vi "svx_Build Data from Magnitude and Phase (N Orders).vi"(5 "reset? (F)":bool, 6 "samples/revolution wanted":i32=4, 7 "samples/revolution":dbl=1.0 format="%.2f", 8 "error in (no error)":errorcluster, 9 "magnitudes info":T1[](array[typedef]) {"x-axis units" items=["Time (s)"=0, "Frequency-CB (Hz)"=1, "Frequency-CPB (Hz)"=1248, "Frequency-Arbitrary (Hz)"=2357, "Quefrency (s)"=2, "Revolutions (rev)"=3, "Order"=4, "Speed (RPM)"=11, "Speed (rad/s)"=21, "Index"=65535]; "weighting filter" items=["Linear", "A-weighting", "B-weighting", "C-weighting", "ITU-R 468-4", "Dolby", "CCITT", "C-message", "Wb", "Wc", "Wd", "We", "Wf", "Wh", "Wj", "Wk", "Wm", "AES17 20 kHz lowpass", "AES17 40 kHz lowpass", "AES17 20 kHz highpass", "AES17 40 kHz highpass"]; "dB reference [EU]" format="%.2f"; "engineering units" items=["custom..."=0, "V"=1, "A"=21, "C"=30, "pC"=31, "s"=32, "-"=29, "Pa"=2, "N"=20, "g"=3, "m/s^2"=4, "m/s"=5, "m"=6, "mm/s"=12, "mm"=13, "micron/s"=14, "micron"=15, "in/s^2"=7, "in/s"=8, "in"=9, "mil/s"=10, "mil"=11, "rad/s^2"=16, "rad/s"=17, "rad"=18, "deg/s^2"=26, "deg/s"=27, "deg"=28, "RPM"=22, "cycle/s^2"=23, "Hz"=24, "cycle"=25, "strain"=19]; "spectral info"."window" items=["None "=0, "Hanning"=1, "Hamming"=2, "Blackman-Harris"=3, "Exact Blackman"=4, "Blackman"=5, "Flat Top"=6, "4 Term B-Harris "=7, "7 Term B-Harris"=8, "Low Sidelobe"=9, "Force - Exponential"=10, "Gaussian"=62]}, 10 "phases [phase lag]":cluster{"time/rev/rpm":dbl[], "phase":dbl[]}[][](array[cluster]) {"phase" format="%.2f"; "time/rev/rpm" format="%.2f"}, 11 "magnitudes [RMS]":T7(array[cluster]) {"magnitude" format="%.2f"; "time/rev/rpm" format="%.2f"}) -> (0 "error out":errorcluster, 2 "actual samples/rev":dbl, 3 "order data":dbl[][][](array[numeric]), 4 "orders to compute":dbl[](array[numeric]))   [LabVIEW 2017]
uses:
  <vilib>/addons/_NISVFA/_Shared subVIs/Controls/svc_Spectrum Info.ctl
  <vilib>/addons/_NISVFA/_Shared subVIs/Controls/svc_X-Axis Units.ctl
  <vilib>/addons/_NISVFA/_Shared subVIs/Controls/svc_Spectrum Type.ctl
  <vilib>/addons/_NISVFA/_Shared subVIs/Controls/svc_Engineering Units Text Ring.ctl
  <vilib>/addons/_NISVFA/_Shared subVIs/Controls/svc_Weighting Filter Text Ring.ctl
  <vilib>/addons/_NISVFA/_Shared subVIs/Controls/svc_Complimentary Spectrum Units.ctl
  <vilib>/Analysis/NI_AALPro.lvlib
  <vilib>/addons/Sound and Vibration/Order Analysis/Resample Order Tracking/SoundVib_Resampling.lvlib
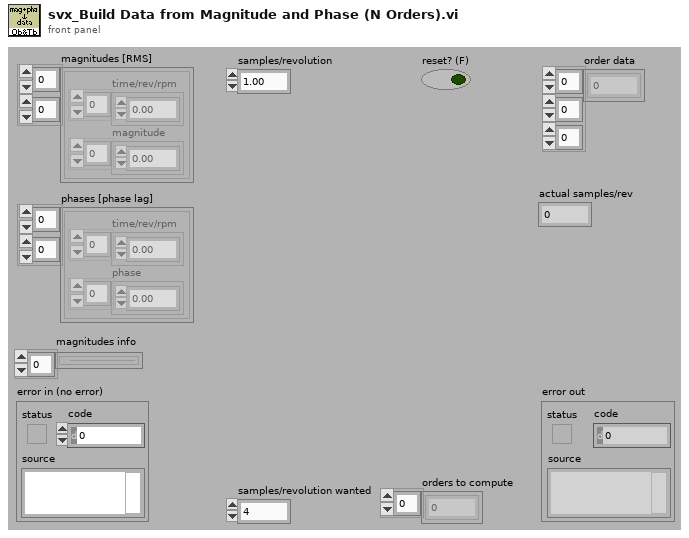
[diagram p1: front panel]
types:
  T1 = typedef "svc_Spectrum Info.ctl" = cluster{"channel name":string, "description":string, "x-axis units":T2, "spectral info":cluster{"spectrum type":T3, "linear/dB":enum16{"linear", "dB"}, "window":u16, "window size":i32, "FFT size":i32}, "engineering units":T4, "custom label":string, "dB reference [EU]":dbl, "peak units":enum16{"rms", "peak", "peak-peak"}, "weighting filter":T5, "spectral density?":bool, "unit label":string, "spectrum skewed?":bool, "complimentary spectrum units":T6}
  T2 = typedef "svc_X-Axis Units.ctl" = u16
  T3 = typedef "svc_Spectrum Type.ctl" = enum16{"FFT Spectrum [complex]", "Amplitude [Magnitude]", "Power [Magnitude^2]", "Cross Spectrum [complex]", "Frequency Response [Complex]"}
  T4 = typedef "svc_Engineering Units Text Ring.ctl" = u16
  T5 = typedef "svc_Weighting Filter Text Ring.ctl" = u16
  T6 = typedef "svc_Complimentary Spectrum Units.ctl" = enum16{"none", "radians", "degrees", "cycles", "imaginary"}
  T7 = cluster{"time/rev/rpm":dbl[], "magnitude":dbl[]}[][]
  T8 = typedef "OAT Decimation Filter.ctl" = cluster{"coefficients":dbl[], "factor":i32}
  T9 = cluster{"dB on? (F)":bool, "unwrap phase? (T)":bool, "unit in degree? (T)":bool}
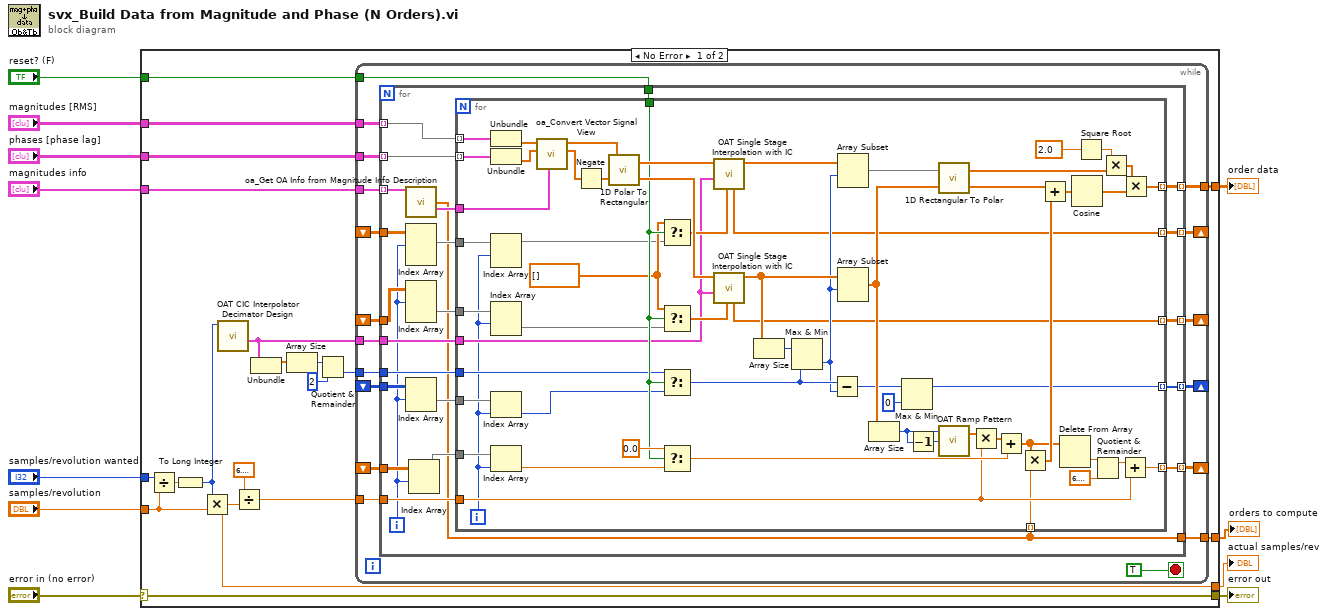
[diagram p0: block diagram]
diagram:
  n1 = case shown="No Error" "error in (no error)" {
    selector: "error in (no error)" -> [w15 w131]
    tunnel: "magnitudes [RMS]" -> [w30 _]
    tunnel: "phases [phase lag]" -> [w29 _]
    tunnel: "reset? (F)" -> [w28 _]
    tunnel: "samples/revolution wanted" -> [w25 _]
    tunnel: "samples/revolution" -> [w24 _]
    tunnel: [w16 _] -> w5
    tunnel: [w15 w131] -> w4
    tunnel: [w14 _] -> w3
    tunnel: "magnitudes info" -> [w13 _]
    tunnel: [w12 _] -> w1
    frame No Error {
      n2 = Divide(x=w25, y=w24) -> (x/y=w27:dbl)
      n3 = To Long Integer(number=w27) -> (32bit integer=w20:i32)
      n4 = Multiply(x=w20, y=w24) -> (x*y=w16:dbl)
      n5 = call <vilib>:"OAT CIC Interpolator Decimator Design.vi"("interpolation/decimation factor"=w20) -> ("filter"=w18:T8)  [unwired: 9 in, 1 out]
      n6 = Divide(x=6.283185307179586, y=w16) -> (x/y=w17:dbl)
      n7 = Unbundle(w18) -> ("coefficients"=w23:dbl[])  [unwired: 1 out]
      n8 = Array Size(array=w23) -> (size(s)=w22:i32)
      n9 = Quotient & Remainder(x=w22, y=2) -> (floor(x/y)=w19:i32)  [unwired: 1 out]
      n10 = while {
        tunnel: w30 -> [w48]
        tunnel: w29 -> [w47]
        tunnel: w28 -> [w46]
        shift-right: [w44] -> _
        shift-left: _ -> [w45]
        shift-right: [w43] -> _
        shift-left: _ -> [w42]
        shift-right: [w41] -> _
        shift-left: _ -> [w40]
        shift-right: [w39] -> _
        shift-left: _ -> [w38]
        tunnel: w19 -> [w37]
        tunnel: w18 -> [w36]
        tunnel: w17 -> [w35]
        tunnel: [w34] -> w14
        tunnel: w13 -> [w32]
        tunnel: [w31] -> w12
        stop <- TRUE stop-if-true
        n11 = for {
          tunnel: w48 -> [w71] mode=indexing
          tunnel: w47 -> [w70] mode=indexing
          tunnel: w46 -> [w69]
          tunnel: w45 -> [w61]
          tunnel: [w68] -> w44 mode=indexing
          tunnel: [w67] -> w43 mode=indexing
          tunnel: w42 -> [w58]
          tunnel: [w66] -> w41 mode=indexing
          tunnel: w40 -> [w56]
          tunnel: [w65] -> w39 mode=indexing
          tunnel: w38 -> [w53]
          tunnel: w37 -> [w57]
          tunnel: w36 -> [w64]
          tunnel: w35 -> [w63]
          tunnel: [w62] -> w34 mode=indexing
          tunnel: w32 -> [w50] mode=indexing
          tunnel: [w51] -> w31
          i -> [w49]
          n12 = call <vilib>:"oa_Get OA Info from Magnitude Info Description.vi"("magnitude info"=w50) -> ("orders to compute"=w51:dbl[], "view"=w52:T9)  [unwired: 10 in, 3 out]
          n13 = Index Array(array=w61, index (dim 0)=w49) -> (element=w60:dbl[][])  [unwired: 2 in]
          n14 = Index Array(array=w58, index (dim 0)=w49) -> (element=w59:dbl[][])  [unwired: 2 in]
          n15 = Index Array(array=w56, index (row)=w49) -> (element=w55:i32[])  [unwired: 1 in]
          n16 = Index Array(array=w53, index (row)=w49) -> (element=w54:dbl[])  [unwired: 1 in]
          n17 = for {
            tunnel: w71 -> [w130] mode=indexing
            tunnel: w70 -> [w129] mode=indexing
            tunnel: w69 -> [w92]
            tunnel: [w91] -> w68 mode=indexing
            tunnel: w60 -> [w82]
            tunnel: [w90] -> w67 mode=indexing
            tunnel: w59 -> [w80]
            tunnel: [w88] -> w66 mode=indexing
            tunnel: w55 -> [w78]
            tunnel: [w87] -> w65 mode=indexing
            tunnel: w54 -> [w76]
            tunnel: w57 -> [w86]
            tunnel: w64 -> [w85]
            tunnel: w63 -> [w84]
            tunnel: [w83] -> w62 mode=indexing
            tunnel: w51 -> [w73] mode=indexing
            tunnel: w52 -> [w72]
            i -> [w74]
            w89 = dbl[] [] ("initial state")
            n18 = Unbundle(w130) -> ("magnitude"=w128:dbl[])  [unwired: 1 out]
            n19 = Unbundle(w129) -> ("phase"=w127:dbl[])  [unwired: 1 out]
            n20 = Index Array(array=w82, index (row)=w74) -> (element=w81:dbl[])  [unwired: 1 in]
            n21 = Index Array(array=w80, index (row)=w74) -> (element=w79:dbl[])  [unwired: 1 in]
            n22 = Index Array(array=w78, index=w74) -> (element=w77:i32)
            n23 = Index Array(array=w76, index=w74) -> (element=w75:dbl)
            n24 = call <vilib>:"oa_Convert Vector Signal View.vi"("view"=w72, "phase"=w127, "magnitude"=w128) -> ("phase out"=w93:dbl[], "magnitude out"=w94:dbl[])  [unwired: 7 in]
            n25 = Negate(x=w93) -> (-x=w108:dbl[])
            n26 = call <vilib>:"1D Polar To Rectangular.vi"("Magnitude"=w94, "Phase"=w108) -> ("X"=w107:dbl[], "Y"=w106:dbl[])  [unwired: 1 out]
            n27 = Select(t=w89, s=w92, f=w81) -> (s? t:f=w105:dbl[])
            n28 = Select(t=w89, s=w92, f=w79) -> (s? t:f=w104:dbl[])
            n29 = Select(t=w86, s=w92, f=w77) -> (s? t:f=w98:i32)
            n30 = Select(t=0.0, s=w92, f=w75) -> (s? t:f=w110:dbl)
            n31 = call <vilib>:"OAT Single Stage Interpolation with IC.vi"("initial state"=w105, "filter"=w85, "X"=w107) -> ("Y"=w103:dbl[], "final state"=w91:dbl[])  [unwired: 6 in, 1 out]
            n32 = call <vilib>:"OAT Single Stage Interpolation with IC.vi"("initial state"=w104, "filter"=w85, "X"=w106) -> ("Y"=w100:dbl[], "final state"=w90:dbl[])  [unwired: 6 in, 1 out]
            n33 = Array Size(array=w100) -> (size(s)=w99:i32)
            n34 = Max & Min(x=w99, y=w98) -> (min(x,y)=w95:i32)  [unwired: 1 out]
            n35 = Subtract(x=w98, y=w95) -> (x-y=w97:i32)
            n36 = Array Subset(array=w103, index=w95) -> (w102:dbl[])  [unwired: 1 in]
            n37 = Array Subset(array=w100, index=w95) -> (w101:dbl[])  [unwired: 1 in]
            n38 = Array Size(array=w101) -> (size(s)=w109:i32)
            n39 = Max & Min(x=w97, y=0) -> (max(x,y)=w88:i32)  [unwired: 1 out]
            n40 = Decrement(x=w109) -> (x-1=w126:i32)
            n41 = call <vilib>:"1D Rectangular To Polar.vi"("X"=w102, "Y"=w101) -> ("Magnitude"=w119:dbl[], "Phase"=w120:dbl[])  [unwired: 1 out]
            n42 = call <vilib>:"OAT Ramp Pattern.vi"("end"=w126, "samples"=w109) -> ("Ramp Pattern"=w118:dbl[])  [unwired: 1 in, 1 out]
            n43 = Multiply(x=w118, y=w84) -> (x*y=w113:dbl[])
            n44 = Add(x=w113, y=w110) -> (x+y=w112:dbl[])
            n45 = Multiply(x=w112, y=w73) -> (x*y=w123:dbl[])
            n46 = Add(x=w120, y=w123) -> (x+y=w122:dbl[])
            n47 = Delete From Array(array=w112) -> (deleted portion=w116:dbl)  [unwired: 2 in, 1 out]
            n48 = Cosine(x=w122) -> (cos(x)=w121:dbl[])
            n49 = Square Root(x=2.0) -> (sqrt(x)=w124:dbl)
            n50 = Quotient & Remainder(x=w116, y=6.283185307179586) -> (x-y*floor(x/y)=w114:dbl)  [unwired: 1 out]
            n51 = Multiply(x=w124, y=w119) -> (x*y=w117:dbl[])
            n52 = Add(x=w114, y=w84) -> (x+y=w87:dbl)
            n53 = Multiply(x=w117, y=w121) -> (x*y=w83:dbl[])
          }
        }
      }
    }
    frame Error {
    }
  }
  "actual samples/rev" <- w5
  "error out" <- w4
  "order data" <- w3
  "orders to compute" <- w1
